vi "Metrolab.vi"(7 "error in (no error)":errorcluster caption="エラー入力（エラーなし）") -> (0 "配列":dbl[](array[numeric]), 3 "error out":errorcluster caption="エラー出力" {"code" format="%.0x"})   [LabVIEW 2017]
panel:
  in  "VISA resource name":refnum<visa-resource-name>="COM5"
  out "String":string="\r\n"
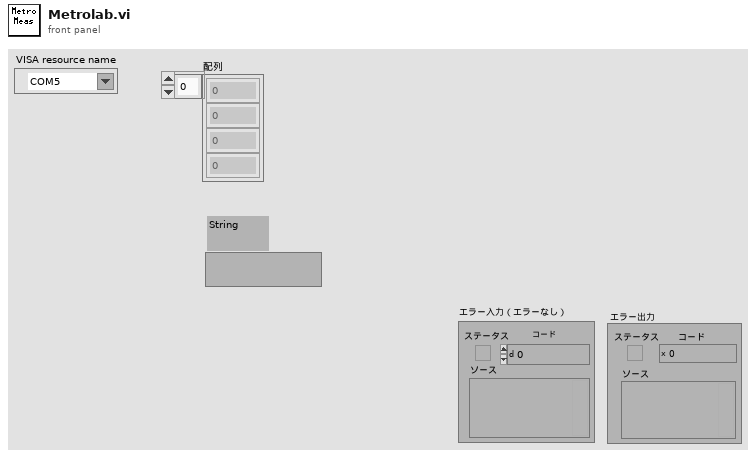
[diagram p1: front panel]
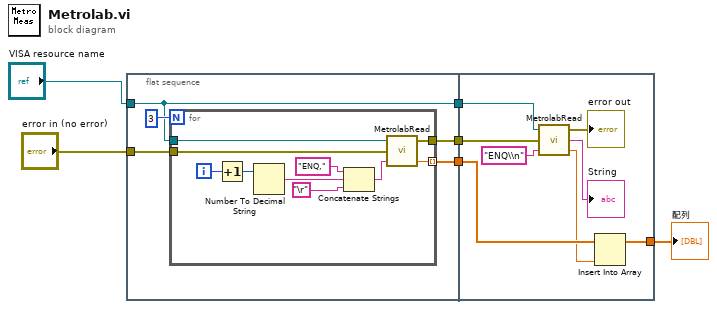
[diagram p0: block diagram]
diagram:
  n1 = flat-sequence {
    tunnel: "VISA resource name" -> [w10]
    tunnel: [w10] -> w5
    tunnel: [w9] -> w4
    tunnel: [w8] -> w3
    tunnel: "error in (no error)" -> [w7]
    tunnel: w5 -> [w29]
    tunnel: w4 -> [w27]
    tunnel: w3 -> [w25]
    tunnel: [w23] -> w2
    frame #0 {
      n2 = for {
        N: 3 -> [_]
        tunnel: w10 -> [w21]
        tunnel: [w17] -> w8 mode=indexing
        tunnel: [w13] -> w9
        tunnel: w7 -> [w12]
        i -> [w14]
        n3 = Increment(x=w14) -> (x+1=w15:i32)
        n4 = Number To Decimal String(number=w15) -> (decimal integer string=w18:string)  [unwired: 1 in]
        n5 = Concatenate Strings("ENQ,", w18, "\r") -> (w19:string)
        n6 = call "MetrolabRead.vi"("Input string"=w19, "error in (no error)"=w12, "VISA resource name"=w21) -> ("B value [mT]"=w17:dbl, "error out"=w13:errorcluster)  [unwired: 1 out]
      }
    }
    frame #1 {
      n7 = call "MetrolabRead.vi"("Input string"="ENQ\\n", "error in (no error)"=w27, "VISA resource name"=w29) -> ("B value [mT]"=w24:dbl, "String"=→"String":string, "error out"=→"error out":errorcluster)
      n8 = Insert Into Array(array=w25, new element=w24) -> (w23:dbl[])  [unwired: 1 in]
    }
  }
  "配列" <- w2
